vi "GEA2 HEWH Standard ERDs.vi"(8 "Error In":errorcluster, 10 "ERD Data Input":T1[](array[typedef]) {"ERD Number" format="%.0x"}, 11 "ERD Data  in":T2 {"ERD Therm Data"."EEV Possition" format="%0.0f"; "ERD Therm Data"."T6" format="%.1f"; "ERD Therm Data"."T2" format="%.1f"; "ERD Therm Data"."T3a" format="%.1f"; "ERD Therm Data"."T3b" format="%.1f"; "ERD Therm Data"."T4" format="%.1f"; "ERD Therm Data"."T5" format="%.1f"; "ERD Therm Data"."Current" format="%.1f"}) -> (0 "Error Out":errorcluster, 2 "ERD Data Output":T1[](array[typedef]) {"ERD Number" format="%.0x"}, 3 "ERD Data  out":T2 {"ERD Therm Data"."EEV Possition" format="%0.0f"; "ERD Therm Data"."T6" format="%.1f"; "ERD Therm Data"."T2" format="%.1f"; "ERD Therm Data"."T3a" format="%.1f"; "ERD Therm Data"."T3b" format="%.1f"; "ERD Therm Data"."T4" format="%.1f"; "ERD Therm Data"."T5" format="%.1f"; "ERD Therm Data"."Current" format="%.1f"})   [LabVIEW 2016]
uses:
  type defs/ERD Read Data Out.ctl
  type defs/HEWH ERD Data.ctl
  type defs/HEWH Faults.ctl
  type defs/HEWH Mixing Valve.ctl
  library/GEA2_Toolkit.lvlib
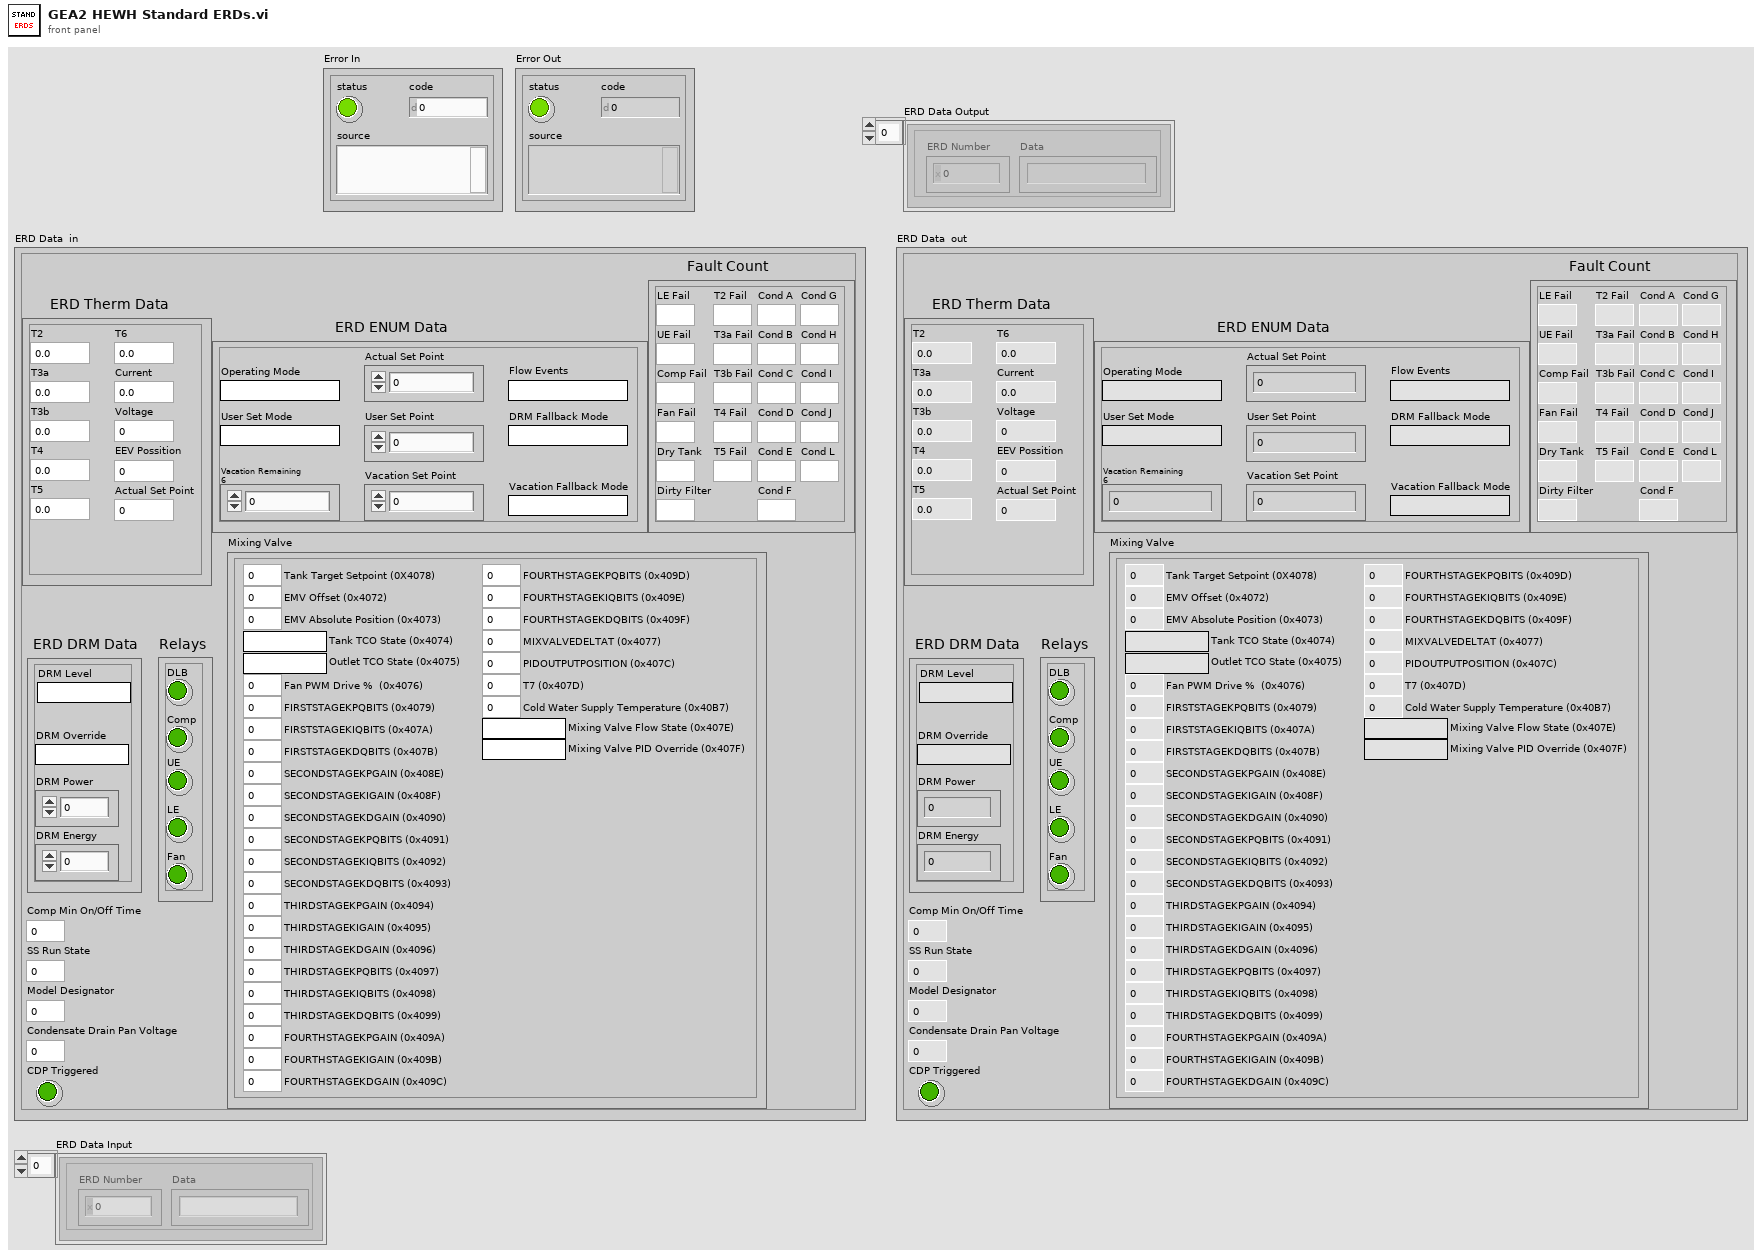
[diagram p1: front panel]
types:
  T1 = typedef "GEA2_Toolkit.lvlib/ERD Read Data Out.ctl" = cluster{"ERD Number":u16, "Data":string}
  T2 = typedef "HEWH ERD Data.ctl" = cluster{"ERD Therm Data":cluster{"T2":dbl, "T3a":dbl, "T3b":dbl, "T4":dbl, "T5":dbl, "T6":dbl, "Current":dbl, "Voltage":dbl, "EEV Possition":dbl, "Actual Set Point":dbl}, "ERD ENUM Data":cluster{"Actual Set Point":dbl, "Flow Events":string, "User Set Mode":string, "Operating Mode":string, "DRM Fallback Mode":string, "Vacation Fallback Mode":string, "User Set Point":dbl, "Vacation Set Point":dbl, "Vacation Remaining\n6":dbl}, "ERD DRM Data":cluster{"DRM Level":string, "DRM Override":string, "DRM Power":dbl, "DRM Energy":dbl}, "Fault Count":T3, "Relays":cluster{"DLB":bool, "Comp":bool, "UE":bool, "LE":bool, "Fan":bool}, "Comp Min On/Off Time":u16, "SS Run State":u16, "Condensate Drain Pan Voltage":u16, "CDP Triggered":bool, "Model Designator":u8, "Mixing Valve":T4}
  T3 = typedef "HEWH Faults.ctl" = cluster{"LE Fail":u32, "UE Fail":u32, "Comp Fail":u32, "T2 Fail":u32, "T3a Fail":u32, "T3b Fail":u32, "T4 Fail":u32, "T5 Fail":u32, "Cond A":u32, "Cond B":u32, "Cond C":u32, "Cond D":u32, "Cond E":u32, "Cond F":u32, "Cond G":u32, "Cond H":u32, "Cond I":u32, "Cond J":u32, "Cond L":u32, "Fan Fail":u32, "Dirty Filter":u32, "Dry Tank":u32}
  T4 = typedef "HEWH Mixing Valve.ctl" = cluster{"Tank Target Setpoint (0X4078)":dbl, "EMV Offset (0x4072)":dbl, "EMV Absolute Position (0x4073)":dbl, "Tank TCO State (0x4074)":string, "Outlet TCO State (0x4075)":string, "Fan PWM Drive %  (0x4076)":dbl, "FIRSTSTAGEKPQBITS (0x4079)":dbl, "FIRSTSTAGEKIQBITS (0x407A)":dbl, "FIRSTSTAGEKDQBITS (0x407B)":dbl, "SECONDSTAGEKPGAIN (0x408E)":dbl, "SECONDSTAGEKIGAIN (0x408F)":dbl, "SECONDSTAGEKDGAIN (0x4090)":dbl, "SECONDSTAGEKPQBITS (0x4091)":dbl, "SECONDSTAGEKIQBITS (0x4092)":dbl, "SECONDSTAGEKDQBITS (0x4093)":dbl, "THIRDSTAGEKPGAIN (0x4094)":dbl, "THIRDSTAGEKIGAIN (0x4095)":dbl, "THIRDSTAGEKDGAIN (0x4096)":dbl, "THIRDSTAGEKPQBITS (0x4097)":dbl, "THIRDSTAGEKIQBITS (0x4098)":dbl, "THIRDSTAGEKDQBITS (0x4099)":dbl, "FOURTHSTAGEKPGAIN (0x409A)":dbl, "FOURTHSTAGEKIGAIN (0x409B)":dbl, "FOURTHSTAGEKDGAIN (0x409C)":dbl, "FOURTHSTAGEKPQBITS (0x409D)":dbl, "FOURTHSTAGEKIQBITS (0x409E)":dbl, "FOURTHSTAGEKDQBITS (0x409F)":dbl, "MIXVALVEDELTAT (0x4077)":dbl, "PIDOUTPUTPOSITION (0x407C)":dbl, "T7 (0x407D)":dbl, "Cold Water Supply Temperature (0x40B7)":dbl, "Mixing Valve Flow State (0x407E)":string, "Mixing Valve PID Override (0x407F)":string}
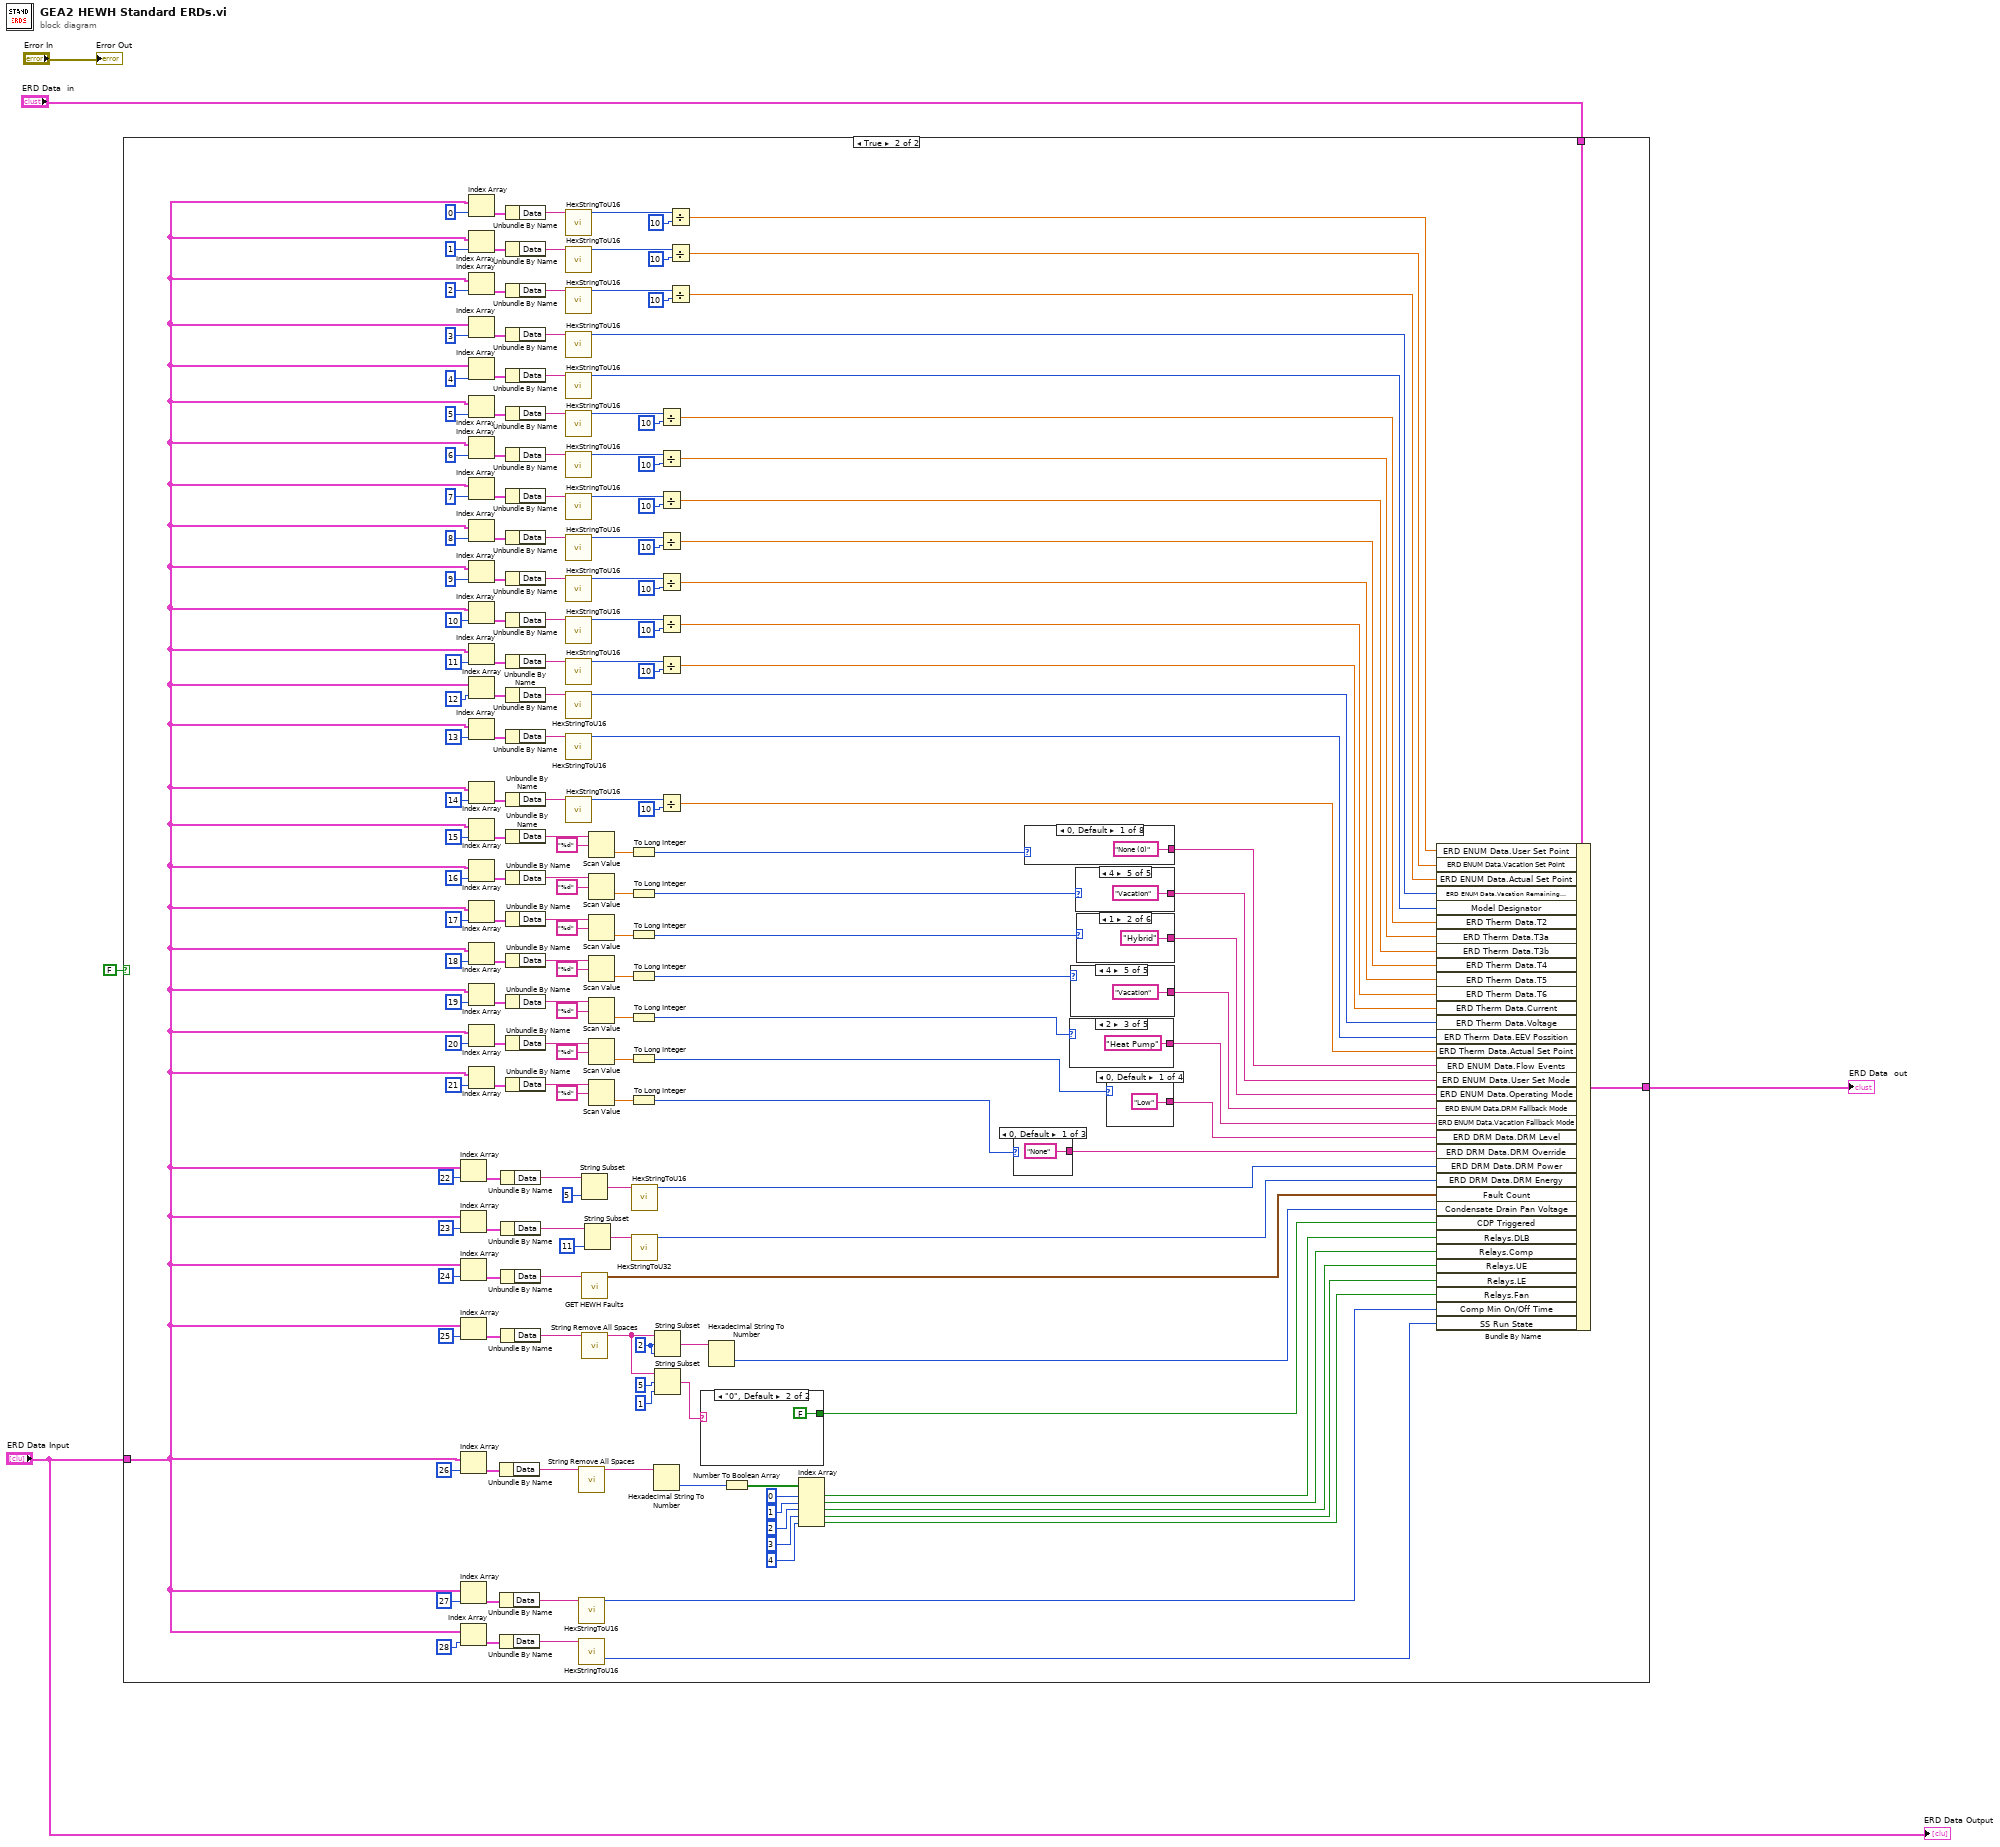
[diagram p0: block diagram]
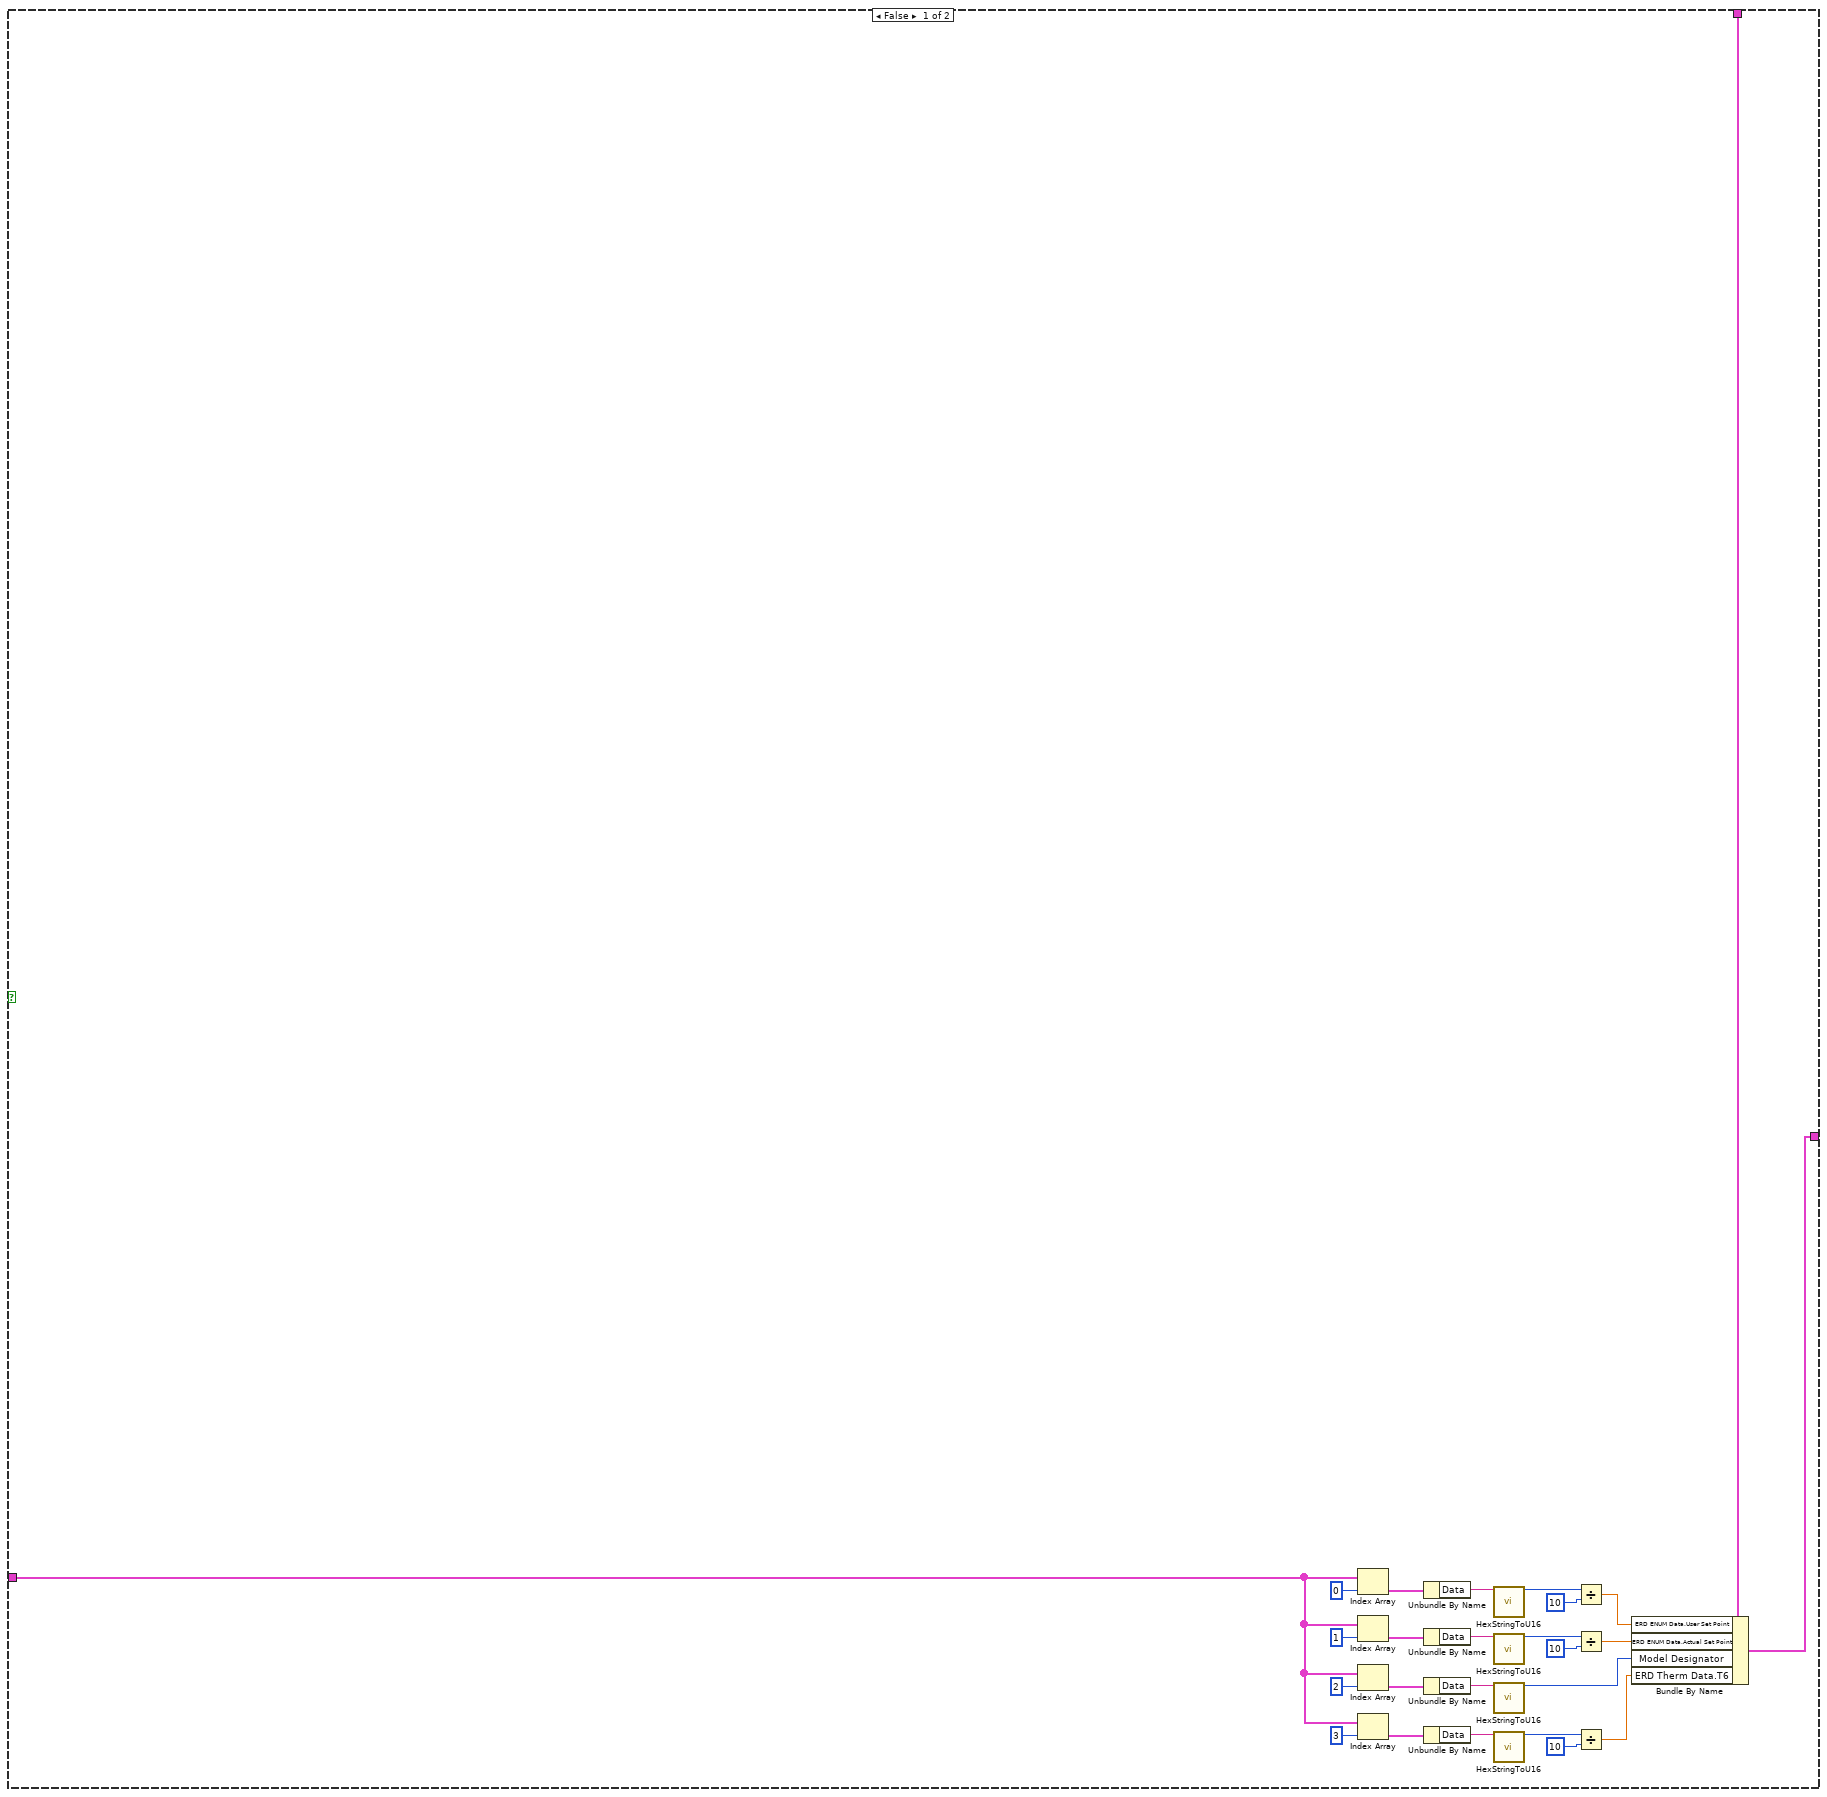
[diagram p2: hidden frame]
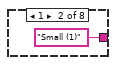
[diagram p3: hidden frame]
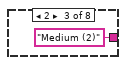
[diagram p4: hidden frame]
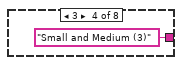
[diagram p5: hidden frame]
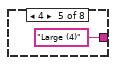
[diagram p6: hidden frame]
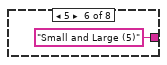
[diagram p7: hidden frame]
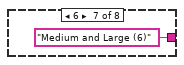
[diagram p8: hidden frame]
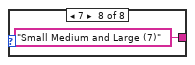
[diagram p9: hidden frame]
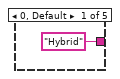
[diagram p10: hidden frame]
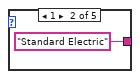
[diagram p11: hidden frame]
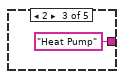
[diagram p12: hidden frame]
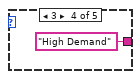
[diagram p13: hidden frame]
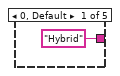
[diagram p14: hidden frame]
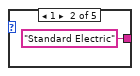
[diagram p15: hidden frame]
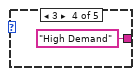
[diagram p16: hidden frame]
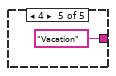
[diagram p17: hidden frame]
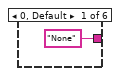
[diagram p18: hidden frame]
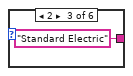
[diagram p19: hidden frame]
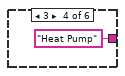
[diagram p20: hidden frame]
diagram:
  n1 = case shown="True" FALSE {
    tunnel: "ERD Data Input" -> [w9 w215]
    tunnel: [w7 w65] -> w4
    tunnel: "ERD Data  in" -> [w6 w64]
    frame False {
      n2 = Index Array(array=w9, index=0) -> (element=w29:T1)
      n3 = Index Array(array=w9, index=1) -> (element=w24:T1)
      n4 = Index Array(array=w9, index=2) -> (element=w18:T1)
      n5 = Index Array(array=w9, index=3) -> (element=w14:T1)
      n6 = Unbundle By Name(w29) -> ("Data"=w30:string)
      n7 = Unbundle By Name(w24) -> ("Data"=w21:string)
      n8 = Unbundle By Name(w18) -> ("Data"=w17:string)
      n9 = Unbundle By Name(w14) -> ("Data"=w11:string)
      n10 = call "HexStringToU16.vi"("Input String"=w30) -> ("Number Out"=w27:u16)  [unwired: 14 in]
      n11 = call "HexStringToU16.vi"("Input String"=w21) -> ("Number Out"=w23:u16)  [unwired: 14 in]
      n12 = call "HexStringToU16.vi"("Input String"=w17) -> ("Number Out"=w15:u16)  [unwired: 14 in]
      n13 = call "HexStringToU16.vi"("Input String"=w11) -> ("Number Out"=w12:u16)  [unwired: 14 in]
      n14 = Divide(x=w27, y=u16 10) -> (x/y=w25:dbl)
      n15 = Divide(x=w23, y=u16 10) -> (x/y=w19:dbl)
      n16 = Divide(x=w12, y=u16 10) -> (x/y=w8:dbl)
      n17 = Bundle By Name(cluster=w6, "ERD ENUM Data.User Set Point"=w25, "ERD ENUM Data.Actual Set Point"=w19, "Model Designator"=w15, "ERD Therm Data.T6"=w8) -> (w7:T2)
    }
    frame True {
      w163 = 2 ("length (rest)")
      n18 = Index Array(array=w215, index=22) -> (element=w152:T1)
      n19 = Index Array(array=w215, index=23) -> (element=w157:T1)
      n20 = Index Array(array=w215, index=24) -> (element=w160:T1)
      n21 = Index Array(array=w215, index=25) -> (element=w169:T1)
      n22 = Index Array(array=w215, index=26) -> (element=w175:T1)
      n23 = Index Array(array=w215, index=27) -> (element=w177:T1)
      n24 = Index Array(array=w215, index=28) -> (element=w180:T1)
      n25 = Index Array(array=w215, index=0) -> (element=w62:T1)
      n26 = Index Array(array=w215, index=1) -> (element=w69:T1)
      n27 = Index Array(array=w215, index=2) -> (element=w75:T1)
      n28 = Index Array(array=w215, index=3) -> (element=w77:T1)
      n29 = Index Array(array=w215, index=4) -> (element=w81:T1)
      n30 = Index Array(array=w215, index=5) -> (element=w86:T1)
      n31 = Index Array(array=w215, index=6) -> (element=w91:T1)
      n32 = Index Array(array=w215, index=7) -> (element=w96:T1)
      n33 = Index Array(array=w215, index=8) -> (element=w101:T1)
      n34 = Index Array(array=w215, index=9) -> (element=w106:T1)
      n35 = Index Array(array=w215, index=10) -> (element=w111:T1)
      n36 = Index Array(array=w215, index=11) -> (element=w116:T1)
      n37 = Index Array(array=w215, index=12) -> (element=w118:T1)
      n38 = Index Array(array=w215, index=13) -> (element=w122:T1)
      n39 = Index Array(array=w215, index=14) -> (element=w127:T1)
      n40 = Index Array(array=w215, index=15) -> (element=w130:T1)
      n41 = Index Array(array=w215, index=16) -> (element=w134:T1)
      n42 = Index Array(array=w215, index=17) -> (element=w137:T1)
      n43 = Index Array(array=w215, index=18) -> (element=w140:T1)
      n44 = Index Array(array=w215, index=19) -> (element=w143:T1)
      n45 = Index Array(array=w215, index=20) -> (element=w146:T1)
      n46 = Index Array(array=w215, index=21) -> (element=w149:T1)
      n47 = Unbundle By Name(w175) -> ("Data"=w176:string)
      n48 = Unbundle By Name(w177) -> ("Data"=w178:string)
      n49 = Unbundle By Name(w180) -> ("Data"=w181:string)
      n50 = Unbundle By Name(w152) -> ("Data"=w153:string)
      n51 = Unbundle By Name(w157) -> ("Data"=w158:string)
      n52 = Unbundle By Name(w160) -> ("Data"=w161:string)
      n53 = Unbundle By Name(w169) -> ("Data"=w170:string)
      n54 = Unbundle By Name(w62) -> ("Data"=w63:string)
      n55 = Unbundle By Name(w69) -> ("Data"=w70:string)
      n56 = Unbundle By Name(w75) -> ("Data"=w72:string)
      n57 = Unbundle By Name(w77) -> ("Data"=w78:string)
      n58 = Unbundle By Name(w81) -> ("Data"=w80:string)
      n59 = Unbundle By Name(w86) -> ("Data"=w83:string)
      n60 = Unbundle By Name(w91) -> ("Data"=w90:string)
      n61 = Unbundle By Name(w96) -> ("Data"=w95:string)
      n62 = Unbundle By Name(w101) -> ("Data"=w98:string)
      n63 = Unbundle By Name(w106) -> ("Data"=w105:string)
      n64 = Unbundle By Name(w111) -> ("Data"=w108:string)
      n65 = Unbundle By Name(w116) -> ("Data"=w115:string)
      n66 = Unbundle By Name(w118) -> ("Data"=w119:string)
      n67 = Unbundle By Name(w122) -> ("Data"=w121:string)
      n68 = Unbundle By Name(w127) -> ("Data"=w124:string)
      n69 = Unbundle By Name(w130) -> ("Data"=w131:string)
      n70 = Unbundle By Name(w134) -> ("Data"=w132:string)
      n71 = Unbundle By Name(w137) -> ("Data"=w136:string)
      n72 = Unbundle By Name(w140) -> ("Data"=w138:string)
      n73 = Unbundle By Name(w143) -> ("Data"=w142:string)
      n74 = Unbundle By Name(w146) -> ("Data"=w144:string)
      n75 = Unbundle By Name(w149) -> ("Data"=w148:string)
      n76 = call "HexStringToU16.vi"("Input String"=w63) -> ("Number Out"=w60:u16)  [unwired: 14 in]
      n77 = call "HexStringToU16.vi"("Input String"=w70) -> ("Number Out"=w68:u16)  [unwired: 14 in]
      n78 = call "HexStringToU16.vi"("Input String"=w72) -> ("Number Out"=w74:u16)  [unwired: 14 in]
      n79 = call "HexStringToU16.vi"("Input String"=w78) -> ("Number Out"=w79:u16)  [unwired: 14 in]
      n80 = call "HexStringToU16.vi"("Input String"=w80) -> ("Number Out"=w82:u16)  [unwired: 14 in]
      n81 = call "HexStringToU16.vi"("Input String"=w83) -> ("Number Out"=w85:u16)  [unwired: 14 in]
      n82 = call "HexStringToU16.vi"("Input String"=w90) -> ("Number Out"=w88:u16)  [unwired: 14 in]
      n83 = call "HexStringToU16.vi"("Input String"=w95) -> ("Number Out"=w94:u16)  [unwired: 14 in]
      n84 = call "HexStringToU16.vi"("Input String"=w98) -> ("Number Out"=w99:u16)  [unwired: 14 in]
      n85 = call "HexStringToU16.vi"("Input String"=w105) -> ("Number Out"=w104:u16)  [unwired: 14 in]
      n86 = call "HexStringToU16.vi"("Input String"=w108) -> ("Number Out"=w109:u16)  [unwired: 14 in]
      n87 = call "HexStringToU16.vi"("Input String"=w115) -> ("Number Out"=w114:u16)  [unwired: 14 in]
      n88 = call "HexStringToU16.vi"("Input String"=w119) -> ("Number Out"=w120:u16)  [unwired: 14 in]
      n89 = call "HexStringToU16.vi"("Input String"=w121) -> ("Number Out"=w123:u16)  [unwired: 14 in]
      n90 = call "HexStringToU16.vi"("Input String"=w124) -> ("Number Out"=w125:u16)  [unwired: 14 in]
      n91 = call "String Remove All Spaces.vi"("Input String"=w176) -> ("Spaces Removed"=w174:string)  [unwired: 13 in, 1 out]
      n92 = call "HexStringToU16.vi"("Input String"=w178) -> ("Number Out"=w179:u16)  [unwired: 14 in]
      n93 = call "HexStringToU16.vi"("Input String"=w181) -> ("Number Out"=w182:u16)  [unwired: 14 in]
      n94 = String Subset(string=w153, length (rest)=5 ("length (rest)")) -> (substring=w150:string)  [unwired: 1 in]
      n95 = call "GET HEWH Faults.vi"("Data"=w161) -> ("Faults"=w162:T3)  [unwired: 10 in]
      n96 = call "String Remove All Spaces.vi"("Input String"=w170) -> ("Spaces Removed"=w166:string)  [unwired: 13 in, 1 out]
      n97 = String Subset(string=w158, length (rest)=11 ("length (rest)")) -> (substring=w155:string)  [unwired: 1 in]
      n98 = Scan Value(string=w131, format string="%d") -> (value=w213:dbl)  [unwired: 1 in, 1 out]
      n99 = Scan Value(string=w132, format string="%d") -> (value=w194:dbl)  [unwired: 1 in, 1 out]
      n100 = Scan Value(string=w136, format string="%d") -> (value=w204:dbl)  [unwired: 1 in, 1 out]
      n101 = Scan Value(string=w138, format string="%d") -> (value=w208:dbl)  [unwired: 1 in, 1 out]
      n102 = Scan Value(string=w142, format string="%d") -> (value=w210:dbl)  [unwired: 1 in, 1 out]
      n103 = Scan Value(string=w144, format string="%d") -> (value=w196:dbl)  [unwired: 1 in, 1 out]
      n104 = Scan Value(string=w148, format string="%d") -> (value=w200:dbl)  [unwired: 1 in, 1 out]
      n105 = To Long Integer(number=w213) -> (32bit integer=w212:i32)
      n106 = To Long Integer(number=w194) -> (32bit integer=w195:i32)
      n107 = To Long Integer(number=w204) -> (32bit integer=w203:i32)
      n108 = To Long Integer(number=w208) -> (32bit integer=w207:i32)
      n109 = To Long Integer(number=w210) -> (32bit integer=w206:i32)
      n110 = To Long Integer(number=w196) -> (32bit integer=w197:i32)
      n111 = To Long Integer(number=w200) -> (32bit integer=w201:i32)
      n112 = call "HexStringToU16.vi"("Input String"=w150) -> ("Number Out"=w154:u16)  [unwired: 14 in]
      n113 = call "HexStringToU32.vi"("Input String"=w155) -> ("Number Out"=w159:u32)  [unwired: 14 in]
      n114 = Hexadecimal String To Number(string=w174) -> (number=w173:u32)  [unwired: 2 in, 1 out]
      n115 = String Subset(string=w166, offset (0)=w163, length (rest)=w163) -> (substring=w168:string)
      n116 = String Subset(string=w166, offset (0)=5, length (rest)=1 ("length (rest)")) -> (substring=w165:string)
      n117 = Divide(x=w85, y=u16 10) -> (x/y=w87:dbl)
      n118 = Divide(x=w88, y=u16 10) -> (x/y=w92:dbl)
      n119 = Divide(x=w94, y=u16 10) -> (x/y=w97:dbl)
      n120 = Divide(x=w99, y=u16 10) -> (x/y=w102:dbl)
      n121 = Divide(x=w104, y=u16 10) -> (x/y=w107:dbl)
      n122 = Divide(x=w109, y=u16 10) -> (x/y=w112:dbl)
      n123 = Divide(x=w114, y=u16 10) -> (x/y=w117:dbl)
      n124 = Divide(x=w125, y=u16 10) -> (x/y=w128:dbl)
      n125 = Divide(x=w60, y=u16 10) -> (x/y=w66:dbl)
      n126 = Divide(x=w68, y=u16 10) -> (x/y=w71:dbl)
      n127 = Divide(x=w74, y=u16 10) -> (x/y=w76:dbl)
      n128 = case shown="\"0\", Default" w165 {
        tunnel: [TRUE FALSE] -> w172
        frame "1" {
        }
        frame "0", Default {
        }
      }
      n129 = Hexadecimal String To Number(string=w168) -> (number=w171:u32)  [unwired: 2 in, 1 out]
      n130 = Number To Boolean Array(number=w173) -> (Boolean array=w183:bool[])
      n131 = Index Array(array=w183, index #1=0 ("index"), index #2=1 ("index"), index #3=2 ("index"), index #4=3 ("index"), index #5=4 ("index")) -> (element #1=w189:bool, element #2=w190:bool, element #3=w191:bool, element #4=w192:bool, element #5=w193:bool)
      n132 = case shown="0, Default" w201 {
        tunnel: ["None" "Partial" "Full"] -> w202
        frame 0, Default {
        }
        frame 1 {
        }
        frame 2 {
        }
      }
      n133 = case shown="0, Default" w212 {
        tunnel: ["None (0)" "Small (1)" "Medium (2)" "Small and Medium (3)" "Large (4)" "Small and Large (5)" "Medium and Large (6)" "Small Medium and Large (7)"] -> w214
        frame 0, Default {
        }
        frame 1 {
        }
        frame 2 {
        }
        frame 3 {
        }
        frame 4 {
        }
        frame 5 {
        }
        frame 6 {
        }
        frame 7 {
        }
      }
      n134 = case shown="2" w206 {
        tunnel: ["Hybrid" "Standard Electric" "Heat Pump" "High Demand" "Vacation"] -> w211
        frame 0, Default {
        }
        frame 1 {
        }
        frame 2 {
        }
        frame 3 {
        }
        frame 4 {
        }
      }
      n135 = case shown="4" w207 {
        tunnel: ["Hybrid" "Standard Electric" "Heat Pump" "High Demand" "Vacation"] -> w209
        frame 0, Default {
        }
        frame 1 {
        }
        frame 2 {
        }
        frame 3 {
        }
        frame 4 {
        }
      }
      n136 = case shown="4" w195 {
        tunnel: ["Hybrid" "Standard Electric" "Heat Pump" "High Demand" "Vacation"] -> w199
        frame 0, Default {
        }
        frame 1 {
        }
        frame 2 {
        }
        frame 3 {
        }
        frame 4 {
        }
      }
      n137 = case shown="1" w203 {
        tunnel: ["None" "Hybrid" "Standard Electric" "Heat Pump" "High Demand" "Vacation"] -> w205
        frame 0, Default {
        }
        frame 1 {
        }
        frame 2 {
        }
        frame 3 {
        }
        frame 4 {
        }
        frame 5 {
        }
      }
      n138 = case shown="0, Default" w197 {
        tunnel: ["Low" "Medium" "High" "Critical"] -> w198
        frame 0, Default {
        }
        frame 1 {
        }
        frame 2 {
        }
        frame 3 {
        }
      }
      n139 = Bundle By Name(cluster=w64, "ERD ENUM Data.User Set Point"=w66, "ERD ENUM Data.Vacation Set Point"=w71, "ERD ENUM Data.Actual Set Point"=w76, "ERD ENUM Data.Vacation Remaining\n6"=w79, "Model Designator"=w82, "ERD Therm Data.T2"=w87, "ERD Therm Data.T3a"=w92, "ERD Therm Data.T3b"=w97, "ERD Therm Data.T4"=w102, "ERD Therm Data.T5"=w107, "ERD Therm Data.T6"=w112, "ERD Therm Data.Current"=w117, "ERD Therm Data.Voltage"=w120, "ERD Therm Data.EEV Possition"=w123, "ERD Therm Data.Actual Set Point"=w128, "ERD ENUM Data.Flow Events"=w214, "ERD ENUM Data.User Set Mode"=w199, "ERD ENUM Data.Operating Mode"=w205, "ERD ENUM Data.DRM Fallback Mode"=w209, "ERD ENUM Data.Vacation Fallback Mode"=w211, "ERD DRM Data.DRM Level"=w198, "ERD DRM Data.DRM Override"=w202, "ERD DRM Data.DRM Power"=w154, "ERD DRM Data.DRM Energy"=w159, "Fault Count"=w162, "Condensate Drain Pan Voltage"=w171, "CDP Triggered"=w172, "Relays.DLB"=w189, "Relays.Comp"=w190, "Relays.UE"=w191, "Relays.LE"=w192, "Relays.Fan"=w193, "Comp Min On/Off Time"=w179, "SS Run State"=w182) -> (w65:T2)
    }
  }
  "ERD Data  out" <- w4
  "Error Out" <- "Error In"
  "ERD Data Output" <- "ERD Data Input"
